vi "test_client.vi"() -> ()   [LabVIEW 2020]
uses:
  Types/http_method_enum.ctl
  Client/Client.lvclass
  Request/Request.lvclass
  ClientBuilder/ClientBuilder.lvclass
  RequestBuilder/RequestBuilder.lvclass
  reqwest.lvlib
panel:
  in  "file":path
  out "is_complete":bool
  out "progress":i32
  in  "Abort":bool
  out "success":bool
  out "string_value 2":string
  out "error out 2":errorcluster
  in  "url":string="https://www.vipm.io"
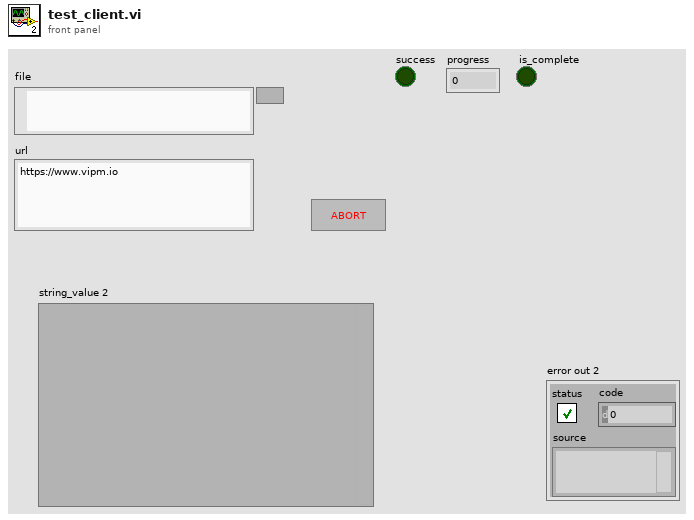
[diagram p1: front panel]
types:
  T1 = typedef "reqwest.lvlib/http_method_enum.ctl" = enum8{"<select>", "GET", "POST", "PUT", "DELETE", "HEAD", "OPTIONS", "CONNECT", "PATCH", "TRACE"}
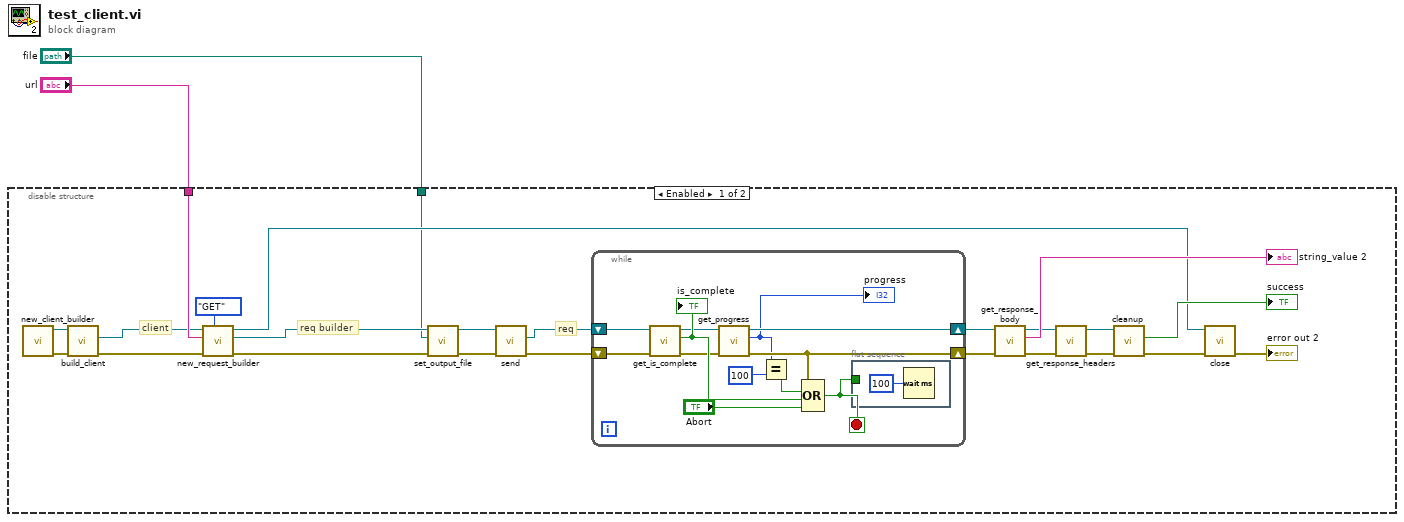
[diagram p0: block diagram]
diagram:
  n1 = disable-structure shown="Enabled" {
    disable-tunnel: "url" -> [w18 _]
    disable-tunnel: "file" -> [w7 _]
    frame Enabled {
      # "req"
      # "req builder"
      # "client"
      n2 = call "new_client_builder.vi"() -> ("error out"=w19:errorcluster, "Client out"=w20:refnum<class "ClientBuilder.lvclass">)  [unwired: 10 in]
      n3 = call "build_client.vi"("error in (no error)"=w19, "ClientBuilder in"=w20) -> ("error out"=w16:errorcluster, "Client out"=w17:refnum<class "Client.lvclass">)  [unwired: 8 in]
      n4 = call "new_request_builder.vi"("HTTP Method"=http_method_enum."GET", "error in (no error)"=w16, "url"=w18, "Client in"=w17) -> ("error out"=w9:errorcluster, "RequestBuilder out"=w12:refnum<class "RequestBuilder.lvclass">, "Client out"=w15:refnum<class "Client.lvclass">)  [unwired: 5 in]
      n5 = call "set_output_file.vi"("error in (no error)"=w9, "output_file"=w7, "obj in"=w12) -> ("error out"=w10:errorcluster, "obj out"=w11:refnum<class "RequestBuilder.lvclass">)  [unwired: 6 in, 1 out]
      n6 = call "send.vi"("error in (no error)"=w10, "obj in"=w11) -> ("error out"=w13:errorcluster, "request"=w14:refnum<class "Request.lvclass">)  [unwired: 8 in]
      n7 = while {
        shift-right: [w33] -> w25
        shift-left: w14 -> [w38]
        shift-right: [w31] -> w24
        shift-left: w13 -> [w37]
        stop <- w27 stop-if-true
        n8 = call "get_is_complete.vi"("error in (no error)"=w37, "Request in"=w38) -> ("error out"=w32:errorcluster, "is_complete"=w36:bool, "Request out"=w34:refnum<class "Request.lvclass">)  [unwired: 7 in]
        "is_complete" <- w36
        n9 = call "get_progress.vi"("error in (no error)"=w32, "Request in"=w34) -> ("error out"=w31:errorcluster, "progress"=w29:i32, "Request out"=w33:refnum<class "Request.lvclass">)  [unwired: 7 in]
        "progress" <- w29
        n10 = Equal?(x=w29, y=100 ("progress")) -> (x = y?=w28:bool)
        n11 = Compound Arithmetic op=OR(w31, w28, w36, "Abort") -> (w27:bool)
        n12 = flat-sequence {
          tunnel: w27 -> [_]
          frame #0 {
            n13 = Wait (ms)(milliseconds to wait=u32 100) -> ()  [unwired: 1 out]
          }
        }
      }
      n14 = call "get_response_body.vi"("error in (no error)"=w24, "Request in"=w25) -> ("error out"=w4:errorcluster, "string_value"=→"string_value 2":string, "Request in"=w6:refnum<class "Request.lvclass">)  [unwired: 7 in]
      n15 = call "get_response_headers.vi"("error in (no error)"=w4, "Request in"=w6) -> ("error out"=w3:errorcluster, "Request in"=w5:refnum<class "Request.lvclass">)  [unwired: 7 in, 1 out]
      n16 = call "cleanup.vi"("error in (no error)"=w3, "Request in"=w5) -> ("error out"=w22:errorcluster, "success"=→"success":bool)  [unwired: 8 in]
      n17 = call "close.vi"("error in (no error)"=w22, "Client in"=w15) -> ("error out"=→"error out 2":errorcluster)  [unwired: 9 in]
    }
    frame Disabled {
    }
  }
